vi "UpdateInstrClass.vi"(8 "error in (no error)":errorcluster caption="entrée d'erreur (pas d'erreur)", 9 "Message":string, 10 "BaseDevice Class":refnum<class "BaseDevice.lvclass">, 11 "Experiment en entrée":refnum<class "Experiment.lvclass"> caption="DNL_LabVIEW Object in") -> (0 "error out":errorcluster caption="sortie d'erreur", 3 "Experiment en sortie":refnum<class "Experiment.lvclass"> caption="DNL_LabVIEW Object out")   [LabVIEW 2019, in "Experiment.lvclass"]
uses:
  Experiment.lvclass
  DevicesClass/BaseDevice/BaseDevice.lvclass
  Experiment.lvclass/Experiment.ctl
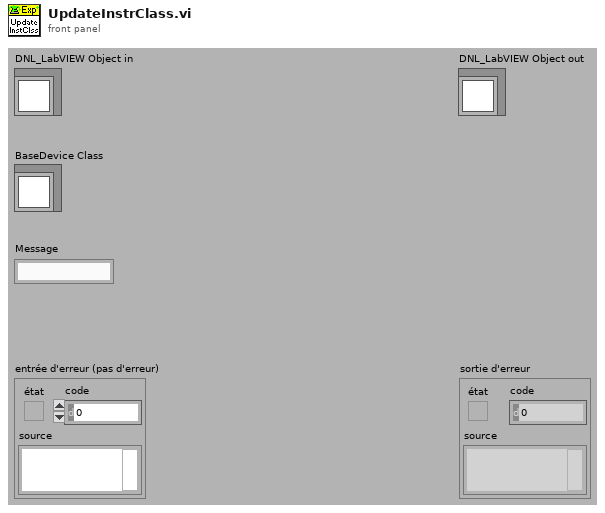
[diagram p1: front panel]
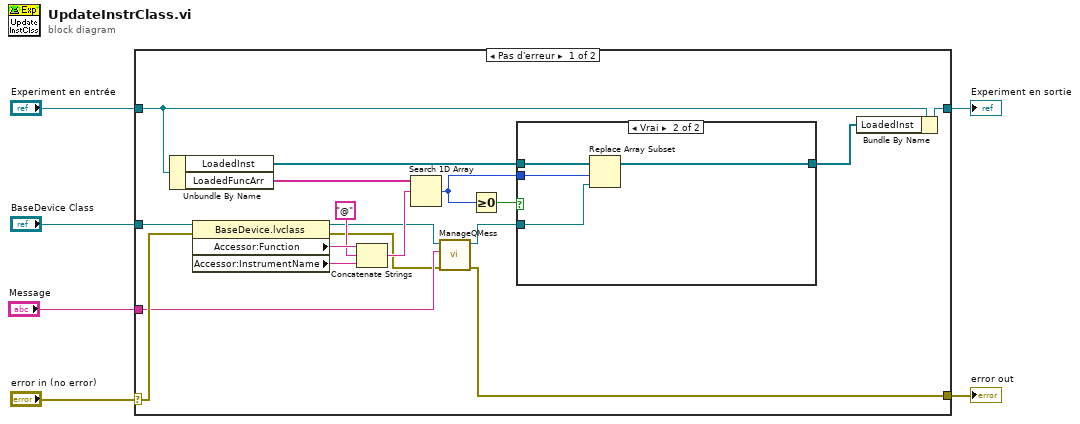
[diagram p0: block diagram]
diagram:
  n1 = case shown="Pas d'erreur" "error in (no error)" {
    selector: "error in (no error)" -> [w18 w31]
    tunnel: [w7 w31] -> w5
    tunnel: [w13 w30] -> w3
    tunnel: "Experiment en entrée" -> [w24 w30]
    tunnel: "BaseDevice Class" -> [w20 _]
    tunnel: "Message" -> [w9 _]
    frame No Error {
      n2 = Unbundle By Name(w24) -> ("LoadedInst"=w16:refnum<class "BaseDevice.lvclass">[], "LoadedFuncArr"=w19:string[])
      n3 = property class="BaseDevice.lvclass"(reference=w20, error in=w18) -> (reference out=w11:refnum<class "BaseDevice.lvclass">, error out=w8:errorcluster, "Accessor:Function"=w23:string, "Accessor:InstrumentName"=w22:string)
      n4 = Concatenate Strings(w23, "@" ("chaîne"), w22) -> (w17:string)
      n5 = Search 1D Array(1D array=w19, element=w17) -> (index of element=w14:i32)  [unwired: 1 in]
      n6 = call-dynamic "ManageQMess.vi"("ErrorIn(No Error)"=w8, "Message"=w9, "BaseDevice.lvclass"=w11) -> ("sortie d'erreur"=w7:errorcluster, "BaseDevice.lvclass Out"=w10:refnum<class "BaseDevice.lvclass">)  [unwired: 7 in]
      n7 = Greater Or Equal To 0?(x=w14) -> (x >= 0?=w15:bool)
      n8 = case shown="Vrai" w15 {
        tunnel: w16 -> [w25 w29]
        tunnel: w10 -> [_ w28]
        tunnel: w14 -> [_ w27]
        tunnel: [w25 w26] -> w12
        frame False {
        }
        frame True {
          n9 = Replace Array Subset(array=w29, new element=w28, index=w27) -> (w26:refnum<class "BaseDevice.lvclass">[])
        }
      }
      n10 = Bundle By Name(cluster=w24, "LoadedInst"=w12) -> (w13:refnum<class "Experiment.lvclass">)
    }
    frame Error {
    }
  }
  "error out" <- w5
  "Experiment en sortie" <- w3
